vi "emi_Convert Bounds to H&W.vi"(2 "Bounds":T1) -> (6 "Width":i32, 7 "Height":i32)   [LabVIEW 2011]
doc: "Use the Bounds cluster(L,T,R,B) in, and get the Width and Height out.\n\n\nSubroutine"
uses:
  <vilib>/Utility/miscctls.llb/LVRectTypeDef.ctl
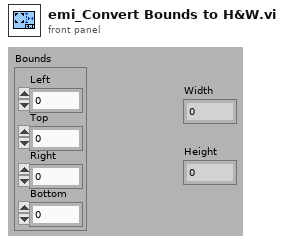
[diagram p1: front panel]
types:
  T1 = typedef "LVRectTypeDef.ctl" = cluster{"Left":i16, "Top":i16, "Right":i16, "Bottom":i16}
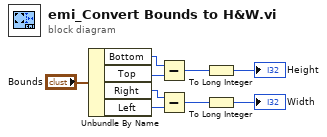
[diagram p0: block diagram]
diagram:
  n1 = Unbundle By Name("Bounds") -> ("Bottom"=w4:i16, "Top"=w5:i16, "Right"=w6:i16, "Left"=w7:i16)
  n2 = Subtract(x=w4, y=w5) -> (x-y=w9:i16)
  n3 = Subtract(x=w6, y=w7) -> (x-y=w8:i16)
  n4 = To Long Integer(number=w9) -> (32bit integer=→"Height":i32)
  n5 = To Long Integer(number=w8) -> (32bit integer=→"Width":i32)
